vi "ULx Write (Digital 2D U32 NChan NSamp).vi"(0 "task in":refnum<k24>, 1 "auto start":bool, 7 "data":u32[][](array[numeric]), 9 "timeout":dbl=10.0 format="%_4g", 11 "error in":errorcluster) -> (4 "task out":refnum<k24>, 10 "number of samples written per channel":u32, 15 "error out":errorcluster)   [LabVIEW 2020]
doc: "Writes one or more 32-bit unsigned integer samples to a task that contains one or more digital output channels. Use an instance that writes 32-bit unsigned integers for devices with up to 32 lines per port."
uses:
  C:/Users/William/Documents/LV 2020 builds/LeaktestDAQ/Source-v33/ULx_LV.dll
  ULx_LV.dll
panel:
  # "channel"
  # "sample #"
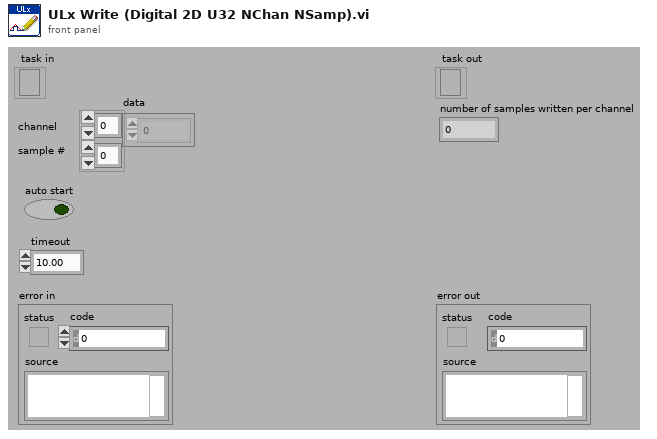
[diagram p1: front panel]
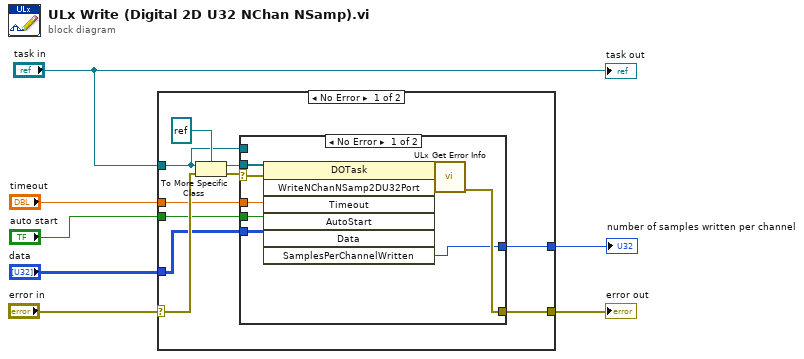
[diagram p0: block diagram]
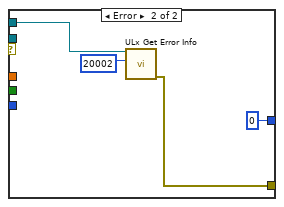
[diagram p2: hidden frame]
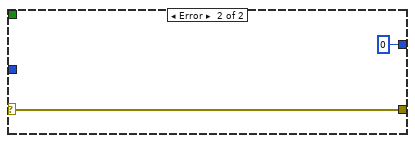
[diagram p3: hidden frame]
diagram:
  n1 = case shown="No Error" "error in" {
    selector: "error in" -> [w17 w33]
    tunnel: "task in" -> [w11 _]
    tunnel: "timeout" -> [w13 _]
    tunnel: [w12 w33] -> w5
    tunnel: "auto start" -> [w10 _]
    tunnel: [w9 0 ("SamplesPerChannelWritten")] -> w2
    tunnel: "data" -> [w8 _]
    frame No Error {
      n2 = To More Specific Class(target class=refnum<k24> refnum, reference=w11, error in=w17) -> (specific class reference=w14:refnum<k24>, error out=w15:errorcluster)
      n3 = case shown="No Error" w15 {
        selector: w15 -> [w26 _]
        tunnel: w14 -> [w27 _]
        tunnel: w13 -> [w20 _]
        tunnel: [w23 w30] -> w12
        tunnel: w11 -> [_ w29]
        tunnel: w10 -> [w19 _]
        tunnel: [w21 0 ("SamplesPerChannelWritten")] -> w9
        tunnel: w8 -> [w18 _]
        frame No Error {
          n4 = invoke class="DOTask" method="WriteNChanNSamp2DU32Port"(reference=w27, error in=w26, "Timeout"=w20, "AutoStart"=w19, "Data"=w18) -> (reference out=w24:refnum<k24>, error out=w25:errorcluster, "WriteNChanNSamp2DU32Port"=w22:i32, "SamplesPerChannelWritten"=w21:u32)  [unwired: 2 in, 3 out]
          n5 = call "ULx Get Error Info.vi"("error in"=w25, "ErrorCode"=w22, "task in"=w24) -> ("error out"=w23:errorcluster)  [unwired: 8 in]
        }
        frame Error {
          n6 = call "ULx Get Error Info.vi"("ErrorCode"=20002, "task in"=w29) -> ("error out"=w30:errorcluster)  [unwired: 9 in]
        }
      }
    }
    frame Error {
    }
  }
  "error out" <- w5
  "number of samples written per channel" <- w2
  "task out" <- "task in"
